vi "libssh2_channel_write.vi"(8 "error in (no error)":errorcluster, 10 "buf":string, 11 "channel":u64) -> (0 "error out":errorcluster, 3 "return value":u64)   [LabVIEW 2013, in "libssh2.lvlib"]
uses:
  libssh2.lvlib
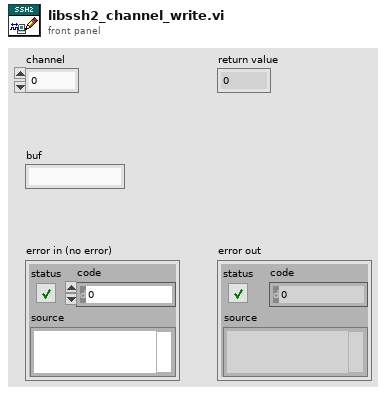
[diagram p1: front panel]
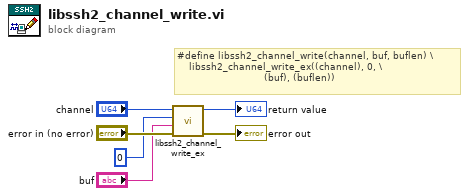
[diagram p0: block diagram]
diagram:
  # "#define libssh2_channel_write(channel, buf, buflen) \\\n    libssh2_channel_write_ex((channel), 0, \\\n                             (buf), (buflen))"
  n1 = call "libssh2_channel_write_ex.vi"("error in (no error)"="error in (no error)", "buf"="buf", "stream_id"=0, "channel"="channel") -> ("error out"=→"error out":errorcluster, "return value"=→"return value":u64)  [unwired: 6 in]
